vi "SectionLocked.vi"(2 "Control Name":string, 3 "DIMControSet (Locks)":refnum<vi>[](array[refnum])) -> (0 "Linked?":bool, 1 "Unlocked?":bool)   [LabVIEW 2014, in "Panels.lvlib"]
uses:
  Panels.lvlib
  Instance           1 21Saved   SectionLocked .vi
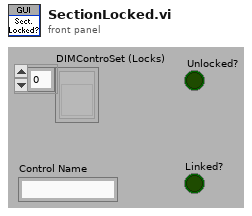
[diagram p1: front panel]
types:
  T1 = cluster{"data":i16, "no link":bool, "quality":i32, "timeStamp":dbl}
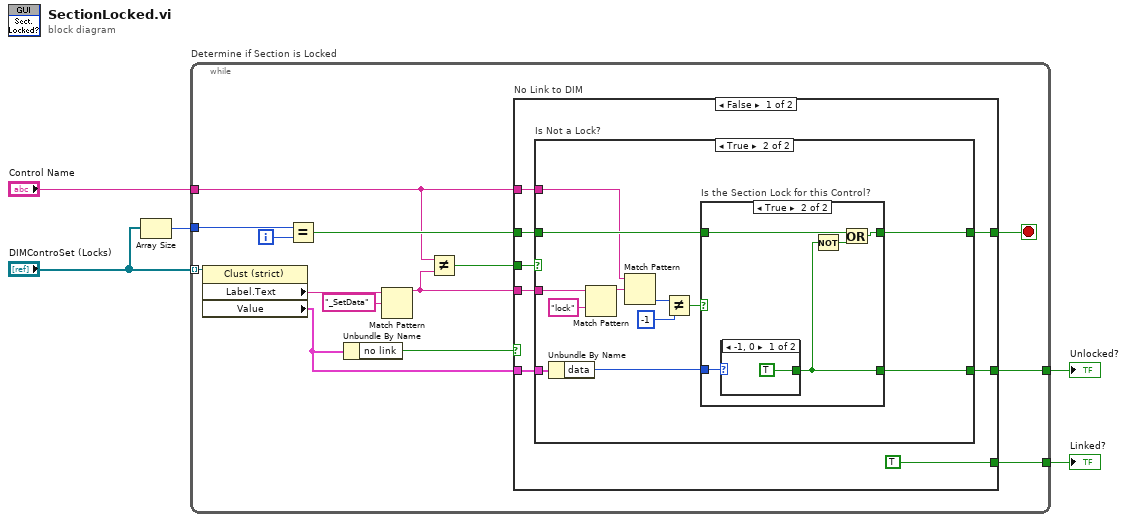
[diagram p0: block diagram]
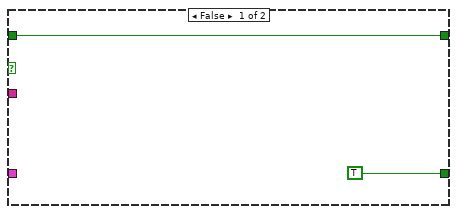
[diagram p2: hidden frame]
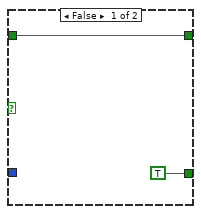
[diagram p3: hidden frame]
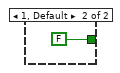
[diagram p4: hidden frame]
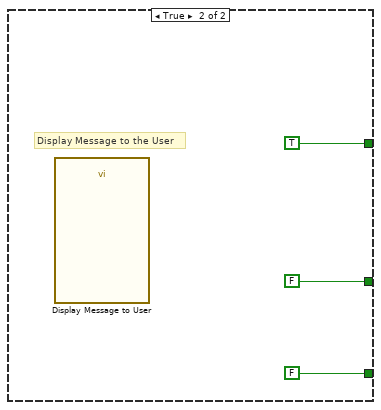
[diagram p5: hidden frame]
diagram:
  n1 = Array Size(array="DIMControSet (Locks)") -> (size(s)=w3:i32)
  n2 = while "Determine if Section is Locked" {
    tunnel: "DIMControSet (Locks)" -> [w19] mode=indexing
    tunnel: "Control Name" -> [w9]
    tunnel: w3 -> [w18]
    tunnel: [w14] -> w2
    tunnel: [w6] -> w1
    i -> [w17]
    stop <- w16 stop-if-true
    n3 = property class="Clust (strict)"(reference=w19) -> ("Label.Text"=w12:string, "Value"=w8:T1)  [unwired: 1 in, 2 out]
    n4 = Equal?(x=w18, y=w17) -> (x = y?=w15:bool)
    n5 = Unbundle By Name(w8) -> ("no link"=w7:bool)
    n6 = Match Pattern(string=w12, regular expression="_SetData") -> (before substring=w10:string)  [unwired: 1 in, 3 out]
    n7 = Not Equal?(x=w9, y=w10) -> (x != y?=w11:bool)
    n8 = case "No Link to DIM" shown="False" w7 {
      tunnel: [w27 TRUE] -> w16
      tunnel: w15 -> [w26 _]
      tunnel: [w25 FALSE] -> w14
      tunnel: w11 -> [w24 _]
      tunnel: w10 -> [w23 _]
      tunnel: w9 -> [w22 _]
      tunnel: w8 -> [w21 _]
      tunnel: [TRUE FALSE] -> w6
      frame False {
        n9 = case "Is Not a Lock?" shown="True" w24 {
          tunnel: w23 -> [_ w41]
          tunnel: w21 -> [_ w39]
          tunnel: [w29 w37] -> w27
          tunnel: w26 -> [w29 w36]
          tunnel: [TRUE w35] -> w25
          tunnel: w22 -> [_ w34]
          frame False {
          }
          frame True {
            n10 = Unbundle By Name(w39) -> ("data"=w38:i16)
            n11 = Match Pattern(string=w41, regular expression="lock") -> (before substring=w33:string)  [unwired: 1 in, 3 out]
            n12 = Match Pattern(string=w34, regular expression=w33) -> (offset past match=w32:i32)  [unwired: 1 in, 3 out]
            n13 = Not Equal?(x=w32, y=-1) -> (x != y?=w30:bool)
            n14 = case "Is the Section Lock for this Control?" shown="True" w30 {
              tunnel: w38 -> [_ w48]
              tunnel: [w43 w47] -> w37
              tunnel: w36 -> [w43 w46]
              tunnel: [TRUE w44] -> w35
              frame False {
              }
              frame True {
                n15 = case shown="-1, 0" w48 {
                  tunnel: [TRUE FALSE] -> w44
                  frame -1, 0 {
                  }
                  frame 1, Default {
                  }
                }
                n16 = Not(x=w44) -> (.not. x?=w45:bool)
                n17 = Or(x=w46, y=w45) -> (x .or. y?=w47:bool)
              }
            }
          }
        }
      }
      frame True {
        # "Display Message to the User"
        n18 = call "Display Message to User"() -> ()  [unwired: 10 in, 2 out]
      }
    }
  }
  "Unlocked?" <- w2
  "Linked?" <- w1
